vi "dfd_FXP Direct IIR I Transposed with IS.vi"(6 "state in":i64[](array[numeric]), 7 "quantizers":T5[](array[typedef]) {"source" items=["Coef a/k"=0, "Coef b/v"=7, "Input"=1, "Output"=2, "Multiplicand"=3, "Product"=4, "Sum"=5, "Delay"=6, "Gain"=8]}, 8 "filtering statistics in":T4(array[cluster]) {"statistics information"."min value" format="%.2f"; "statistics information"."max value" format="%.2f"; "Quantizer Source" items=["Coefficients a/k"=0, "Coefficients b/v"=7, "Input"=1, "Output"=2, "Multiplicand"=3, "Product"=4, "Sum"=5, "Delay"=6]}, 9 "coef a":T7, 10 "coef b":T7, 11 "X":T7) -> (0 "filtering statistics out":T4(array[cluster]) {"statistics information"."min value" format="%.2f"; "statistics information"."max value" format="%.2f"; "Quantizer Source" items=["Coefficients a/k"=0, "Coefficients b/v"=7, "Input"=1, "Output"=2, "Multiplicand"=3, "Product"=4, "Sum"=5, "Delay"=6]}, 3 "filtered X":T7, 4 "state out":i64[](array[numeric]))   [LabVIEW 2017, in "NI_DigFilter_FXP.lvlib"]
uses:
  <vilib>/addons/Digital Filter Design/NI_DigFilter_FXP.lvlib
  <vilib>/addons/Digital Filter Design/_Objects.llb/dfd_DFXP Data Type (vector).ctl
  <vilib>/addons/Digital Filter Design/_Objects.llb/dfd_DFXP Operation Parameter.ctl
  <vilib>/addons/Digital Filter Design/_Objects.llb/dfd_Internal Quantization Srcs.ctl
  <vilib>/addons/Digital Filter Design/_Objects.llb/DFD Quantization Sources.ctl
  <vilib>/addons/Digital Filter Design/_Objects.llb/DFD FXP Statistics Data.ctl
  <vilib>/addons/Digital Filter Design/_Objects.llb/dfd_DFXP Data Type (scaler).ctl
  <vilib>/addons/Digital Filter Design/NI_DigFilterLicensed.lvlib
panel:
  in  "DFXP Value":T1={"value"=0, "wl"=0, "iwl"=0, "Signed"=TRUE} {"value" format="%.0x"}
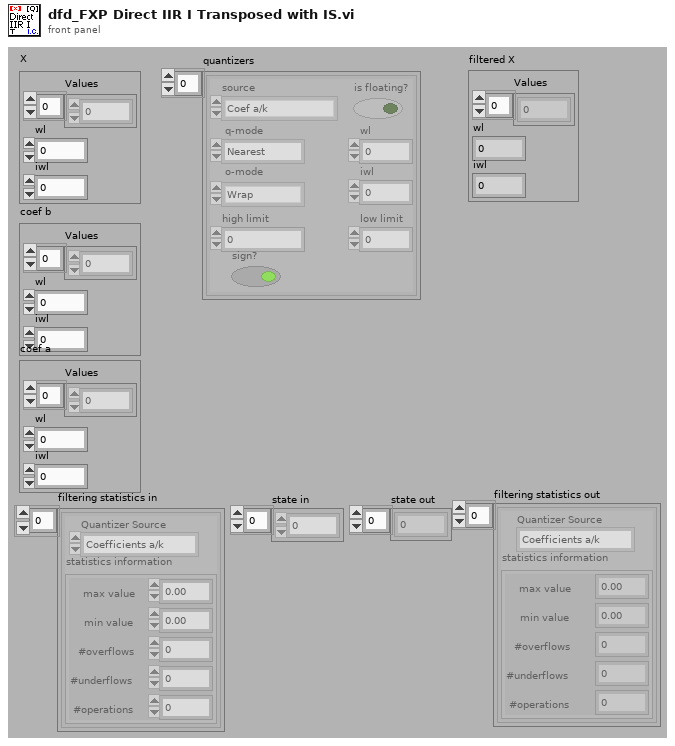
[diagram p1: front panel]
types:
  T1 = typedef "dfd_DFXP Data Type (scaler).ctl" = cluster{"value":i64, "wl":i16, "iwl":i16, "Signed":bool}
  T2 = typedef "NI_DigFilterLicensed.lvlib/DFD Quantization Sources.ctl" = u16
  T3 = typedef "NI_DigFilterLicensed.lvlib/DFD FXP Statistics Data.ctl" = cluster{"max value":ext, "min value":ext, "#overflows":i32, "#underflows":i32, "#operations":i32}
  T4 = cluster{"Quantizer Source":T2, "statistics information":T3}[]
  T5 = typedef "dfd_DFXP Operation Parameter.ctl" = cluster{"source":T6, "is floating?":bool, "o-mode":enum16{"Saturation", "Wrap"}, "q-mode":enum16{"Nearest", "Truncation"}, "wl":i16, "high limit":i64, "low limit":i64, "iwl":i16, "sign?":bool}
  T6 = typedef "NI_DigFilterLicensed.lvlib/dfd_Internal Quantization Srcs.ctl" = u16
  T7 = typedef "dfd_DFXP Data Type (vector).ctl" = cluster{"Values":i64[], "wl":i16, "iwl":i16}
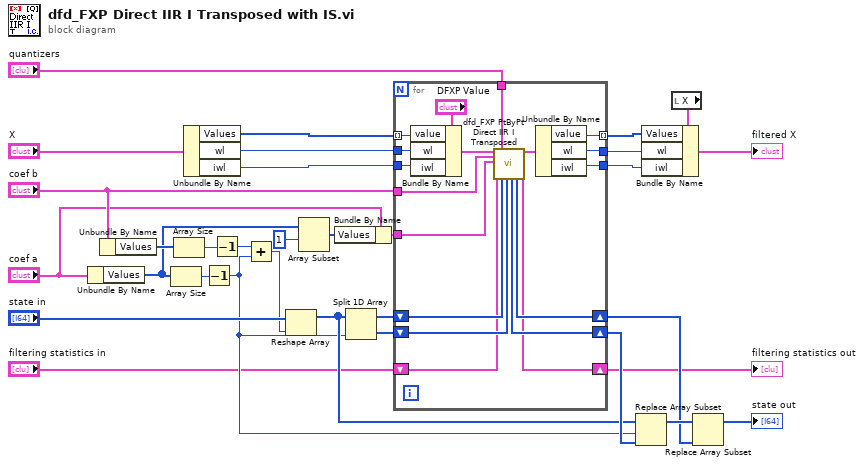
[diagram p0: block diagram]
diagram:
  n1 = Unbundle By Name("coef a") -> ("Values"=w10:i64[])
  n2 = Unbundle By Name("coef b") -> ("Values"=w11:i64[])
  n3 = Array Size(array=w10) -> (size(s)=w30:i32)
  n4 = Array Size(array=w11) -> (size(s)=w32:i32)
  n5 = Unbundle By Name("X") -> ("Values"=w7:i64[], "wl"=w6:i16, "iwl"=w5:i16)
  n6 = Decrement(x=w30) -> (x-1=w14:i32)
  n7 = Decrement(x=w32) -> (x-1=w27:i32)
  n8 = Add(x=w27, y=w14) -> (x+y=w28:i32)
  n9 = Reshape Array("state in", w28) -> (w15:i64[])
  n10 = Array Subset(array=w10, index=1) -> (w23:i64[])  [unwired: 1 in]
  n11 = Bundle By Name(cluster="coef a", "Values"=w23) -> (w9:T7)
  n12 = Split 1D Array(array=w15, index=w14) -> (first subarray=w26:i64[], second subarray=w25:i64[])
  n13 = for {
    tunnel: w7 -> [w50] mode=indexing
    tunnel: "coef b" -> [w47]
    shift-right: [w42] -> w17
    shift-left: w26 -> [w45]
    shift-right: [w43] -> w19
    shift-left: w25 -> [w44]
    tunnel: w9 -> [w46]
    tunnel: [w35] -> w21 mode=indexing
    tunnel: "quantizers" -> [w48]
    shift-right: [w40] -> w12
    shift-left: "filtering statistics in" -> [w41]
    tunnel: w6 -> [w37]
    tunnel: w5 -> [w36]
    tunnel: [w34] -> w2
    tunnel: [w33] -> w1
    n14 = Bundle By Name(cluster="DFXP Value", "value"=w50, "wl"=w37, "iwl"=w36) -> (w39:T1)
    n15 = call <vilib>:"dfd_FXP PtByPt Direct IIR I Transposed.vi"("x"=w39, "coef b[0..M]"=w47, "coef a[1..N]"=w46, "filtering statistics in"=w41, "quantizers"=w48, "xState in"=w45, "yState in"=w44) -> ("yState out"=w43:i64[], "xState out"=w42:i64[], "filtered x"=w49:T1, "filtering statistics out"=w40:T4)  [unwired: 9 out]
    n16 = Unbundle By Name(w49) -> ("value"=w35:i64, "wl"=w34:i16, "iwl"=w33:i16)
  }
  "filtering statistics out" <- w12
  n17 = Replace Array Subset(array=w15, new element=w19, index=w14) -> (w18:i64[])
  n18 = local read "X"() -> (w3:T7)
  n19 = Bundle By Name(cluster=w3, "Values"=w21, "wl"=w2, "iwl"=w1) -> (→"filtered X":T7)
  n20 = Replace Array Subset(array=w18, new element=w17) -> (→"state out":i64[])  [unwired: 1 in]
